vi "FGV Map DeInit (Do Not Use).vi"(8 "error in":errorcluster) -> (0 "error out":errorcluster)   [LabVIEW 2020, in "FGV Map.lvlib"]
uses:
  FGV Map.lvlib
  Controls/FGV Map Core State.ctl
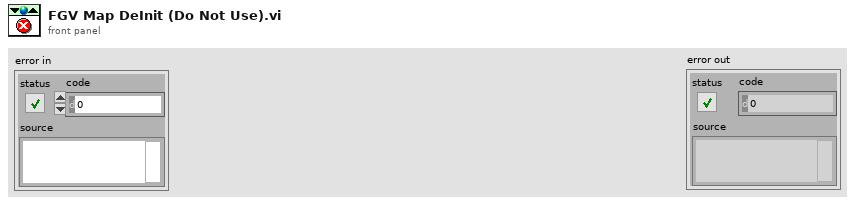
[diagram p1: front panel]
types:
  T1 = typedef "FGV Map.lvlib/FGV Map Core State.ctl" = enum16{"Init", "Set Instance (Unlock)", "Get Instance", "Get Instance (Lock)", "Unlock", "Get All Instances", "Delete Instance"}
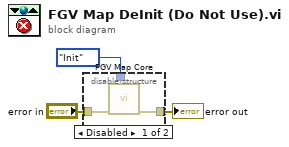
[diagram p0: block diagram]
diagram:
  n1 = disable-structure shown="Disabled" {
    disable-tunnel: FGV_Map_Core_State."Init" ("FGV State") -> [w6 _]
    disable-tunnel: "error in" -> [w5 w7]
    disable-tunnel: [w4 w7] -> w1
    frame Disabled {
      n2 = call "FGV Map Core.vi"("FGV State"=w6, "error in"=w5) -> ("error out"=w4:errorcluster)  [unwired: 5 in, 4 out]
    }
    frame Enabled {
    }
  }
  "error out" <- w1
